vi "Write Pattern Name.vi"(8 "error in (no error)":errorcluster, 10 "Pattern Name":string, 11 "SPI Root Pattern Creator in":refnum<class "SPI Root Pattern Creator.lvclass">) -> (0 "error out":errorcluster, 3 "SPI Root Pattern Creator out":refnum<class "SPI Root Pattern Creator.lvclass">)   [LabVIEW 2018, in "SPI Root Pattern Creator.lvlib" / "SPI Root Pattern Creator.lvclass"]
uses:
  SPI Root Pattern Creator.lvclass
  SPI Root Pattern Creator.lvclass/SPI Root Pattern Creator.ctl
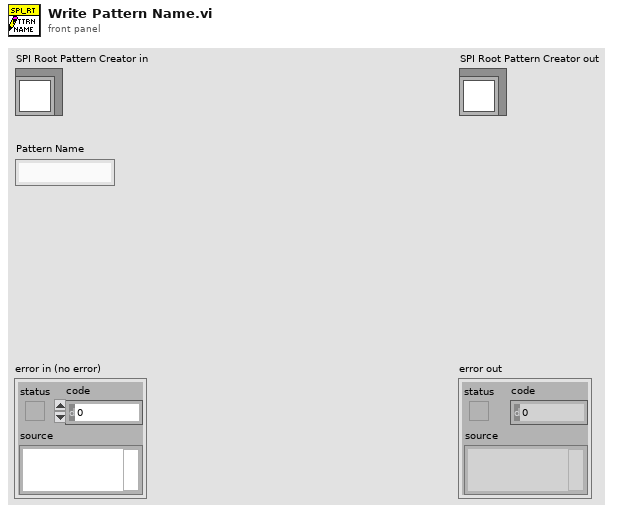
[diagram p1: front panel]
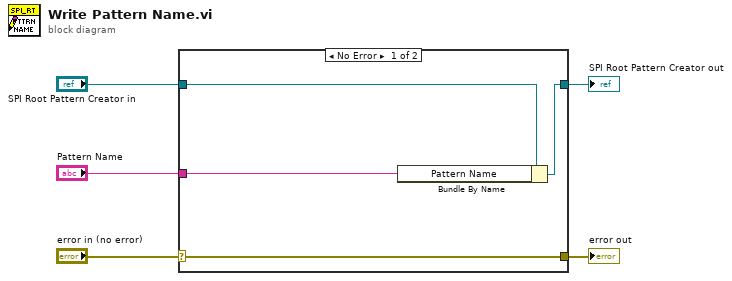
[diagram p0: block diagram]
diagram:
  n1 = case shown="No Error" "error in (no error)" {
    selector: "error in (no error)" -> [w9 w10]
    tunnel: [w9 w10] -> w4
    tunnel: [w7 w11] -> w2
    tunnel: "SPI Root Pattern Creator in" -> [w8 w11]
    tunnel: "Pattern Name" -> [w6 _]
    frame No Error {
      n2 = Bundle By Name(cluster=w8, "Pattern Name"=w6) -> (w7:refnum<class "SPI Root Pattern Creator.lvclass">)
    }
    frame Error {
    }
  }
  "error out" <- w4
  "SPI Root Pattern Creator out" <- w2
